vi "Digital_Output_4Channels.vi"(1 "States":bool[](array[boolean])=[FALSE, FALSE, FALSE, FALSE], 2 "IO":T1={"DO 0"="Mod1/DIO2", "DO 1"="Mod1/DIO2", "DO 2"="Mod1/DIO2", "DO 3"="Mod1/DIO2"}) -> ()   [LabVIEW 2015]
uses:
  <vilib>/rvi/eio/common/nirviEmuTemplateMethod_errors.vi
  <vilib>/eio/EIONode/EIONode.xnode
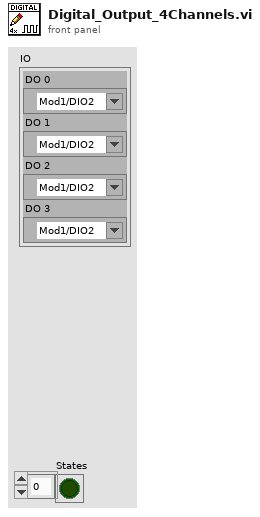
[diagram p1: front panel]
types:
  T1 = cluster{"DO 0":refnum<k21>, "DO 1":refnum<k21>, "DO 2":refnum<k21>, "DO 3":refnum<k21>}
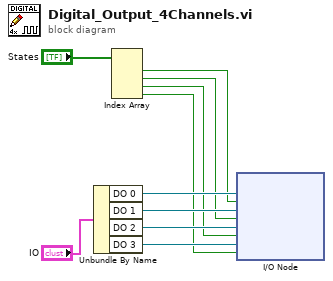
[diagram p0: block diagram]
diagram:
  n1 = Unbundle By Name("IO") -> ("DO 0"=w9:refnum<k21>, "DO 1"=w8:refnum<k21>, "DO 2"=w7:refnum<k21>, "DO 3"=w6:refnum<k21>)
  n2 = Index Array(array="States") -> (element #1=w4:bool, element #2=w3:bool, element #3=w2:bool, element #4=w1:bool)  [unwired: 4 in]
  n3 = xnode "I/O Node"("I/O Item"=w4, "FPGA I/O In"=w9, "I/O Item"=w3, "FPGA I/O In"=w8, "I/O Item"=w2, "FPGA I/O In"=w7, "I/O Item"=w1, "FPGA I/O In"=w6) -> ()  [unwired: 4 out]
